vi "设置指定通道的测频基准脉冲周期.vi"(8 "错误输入":errorcluster caption="错误输入（无错误）", 9 "freqBase_ms":dbl, 10 "chNo":i32, 11 "设备句柄入":i32) -> (0 "错误输出":errorcluster, 1 "real_ms":dbl, 3 "设备句柄":i32=1)   [LabVIEW 2016]
uses:
  dll/em9636.dll
panel:
  in  "超时毫秒":i32=1000
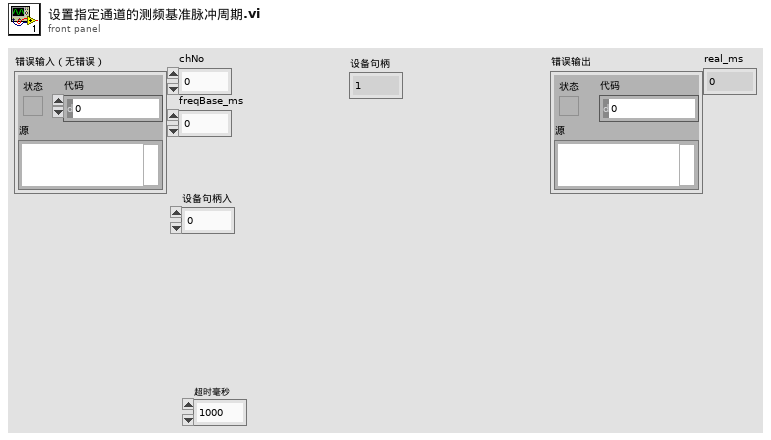
[diagram p1: front panel]
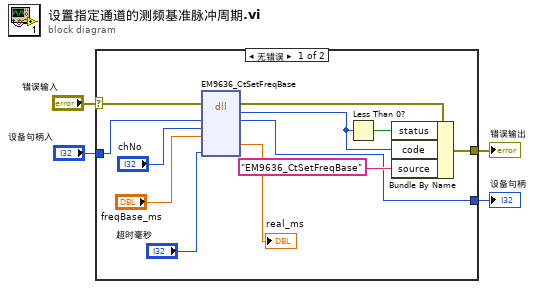
[diagram p0: block diagram]
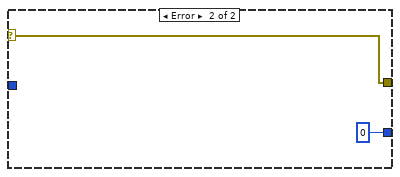
[diagram p2: hidden frame]
diagram:
  n1 = case shown="无错误" "错误输入" {
    selector: "错误输入" -> [w16 w18]
    tunnel: [w12 w18] -> w3
    tunnel: [w8 0 ("错误")] -> w2
    tunnel: "设备句柄入" -> [w10 _]
    frame No Error {
      n2 = dll-call lib="PTH2|abs CUsers\nAdministratorDesktopEM9636original - 副本*EM9636系列_demo_labview(调用DLL方式)dll\nem9636.dll" fn="EM9636_CtSetFreqBase"(error in=w16, "设备句柄"=w10, "chNo"="chNo", "freqBase_ms"="freqBase_ms", "超时毫秒"="超时毫秒") -> (error out=w14:errorcluster, "错误"=w11:i32, "设备句柄"=w8:i32, "real_ms"=→"real_ms":dbl)  [unwired: 6 in, 1 out]
      n3 = Less Than 0?(x=w11) -> (x < 0?=w13:bool)
      n4 = Bundle By Name(cluster=w14, "status"=w13, "code"=w11, "source"="EM9636_CtSetFreqBase") -> (w12:errorcluster)
    }
    frame Error {
    }
  }
  "错误输出" <- w3
  "设备句柄" <- w2
